vi "Write Origin Top.vi"(8 "error in (no error)":errorcluster, 10 "Top":i16, 11 "Picture.lvclass in":refnum<class "Picture.lvclass">) -> (0 "error out":errorcluster, 3 "Picture.lvclass out":refnum<class "Picture.lvclass">)   [LabVIEW 2015, in "Picture.lvclass"]
uses:
  Picture.lvclass
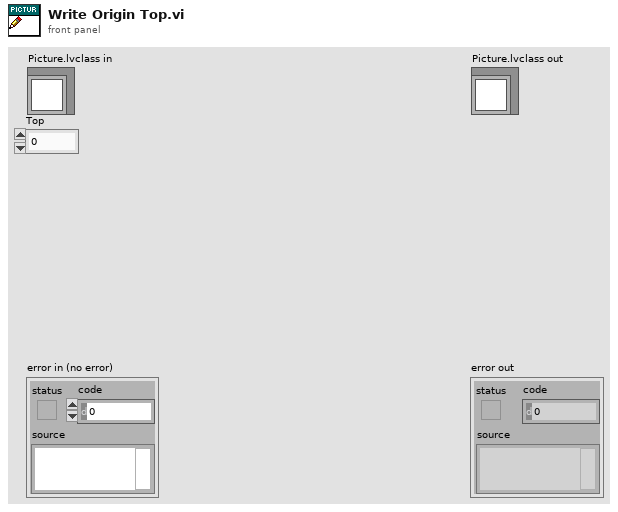
[diagram p1: front panel]
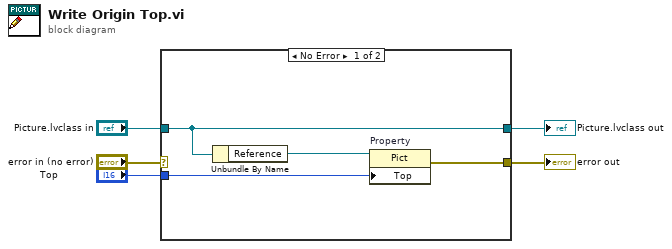
[diagram p0: block diagram]
diagram:
  n1 = case shown="No Error" "error in (no error)" {
    selector: "error in (no error)" -> [_ w11]
    tunnel: [w9 w11] -> w4
    tunnel: [w7 w10] -> w2
    tunnel: "Picture.lvclass in" -> [w7 w10]
    tunnel: "Top" -> [w8 _]
    frame No Error {
      n2 = Unbundle By Name(w7) -> ("Reference"=w6:refnum<vi>)
      n3 = property on="Property" class="Pict"(reference=w6, "Top"=w8) -> (error out=w9:errorcluster)  [unwired: 1 in, 1 out]
    }
    frame Error {
    }
  }
  "error out" <- w4
  "Picture.lvclass out" <- w2
